vi "Set Initialization Data - ConfigView.vi"(8 "error in":errorcluster, 11 "Manager Panel in":refnum<class "Manager Panel.lvclass">) -> (0 "error out":errorcluster, 3 "Manager Panel out":refnum<class "Manager Panel.lvclass">)   [LabVIEW 2020, in "Manager Panel.lvclass"]
doc: "In this VI you can set the initialization data of a statically-linked subWorker."
uses:
  Manager Panel.lvclass
  ConfigView/Initialization Data.ctl
  ConfigView/Response Cases.ctl
  Manager Panel.lvclass/Manager Panel.ctl
  ConfigView/ConfigView.lvclass
  C:/Program Files (x86)/National Instruments/LabVIEW 2020/vi.lib/addons/_Workers/Library/Classes/Worker/Worker.lvclass
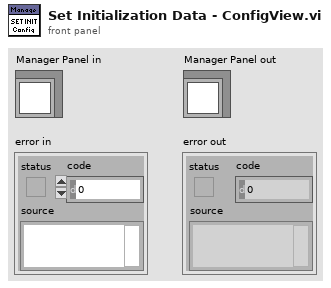
[diagram p1: front panel]
types:
  T1 = typedef "ConfigView.lvclass/Initialization Data.ctl" = cluster{"Response Cases":T2}
  T2 = typedef "ConfigView.lvclass/Response Cases.ctl" = cluster{"Placeholder - Can be deleted":string}
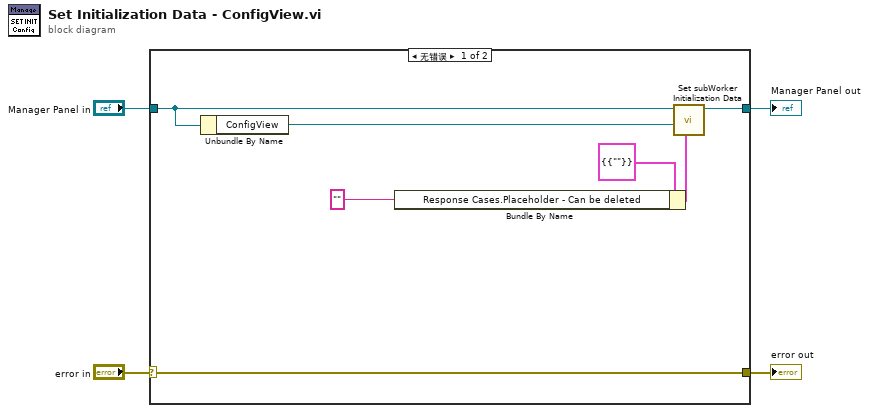
[diagram p0: block diagram]
diagram:
  n1 = case shown="无错误" "error in" {
    selector: "error in" -> [w11 w13]
    tunnel: [w11 w13] -> w3
    tunnel: [w9 w12] -> w2
    tunnel: "Manager Panel in" -> [w8 w12]
    frame No Error {
      n2 = Unbundle By Name(w8) -> ("ConfigView"=w10:refnum<class "ConfigView.lvclass">)
      n3 = Bundle By Name(cluster=T1 {"Response Cases"={"Placeholder - Can be deleted"=""}} ("Initialization Data"), "Response Cases.Placeholder - Can be deleted"="" ("Placeholder")) -> (w6:T1)
      n4 = call-dynamic "Set subWorker Initialization Data.vi"("Initialization Data"=w6, "subWorker"=w10, "Worker"=w8) -> ("Worker out"=w9:refnum<class "Manager Panel.lvclass">)  [unwired: 8 in]
    }
    frame Error {
    }
  }
  "error out" <- w3
  "Manager Panel out" <- w2
